vi "XYGraph.CreateErrorBars.vi"(0 "X":dbl[](array[numeric]) format="%.2f", 5 "Y":dbl[](array[numeric]) format="%.2f", 7 "error low":dbl[](array[numeric]) format="%.2f", 9 "error high":dbl[](array[numeric]) format="%.2f") -> (4 "xy graph bin 2":cluster{"X":dbl[], "Y":dbl[]}[](graph))   [LabVIEW 2013]
doc: "Creates a error bar plot\n\nwww.sciware.com.au"
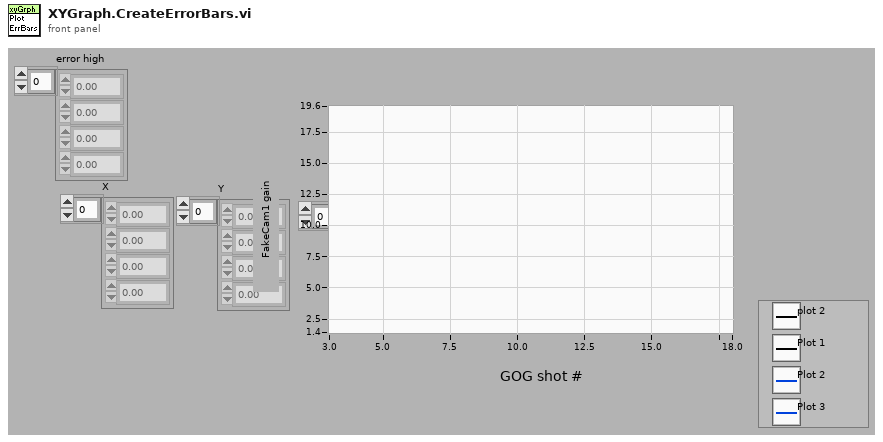
[diagram p1: front panel]
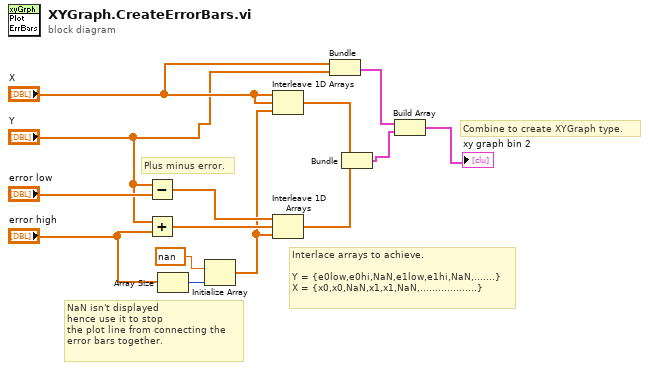
[diagram p0: block diagram]
diagram:
  # "Combine to create XYGraph type."
  # "Interlace arrays to achieve.\n\nY = {e0low,e0hi,NaN,e1low,e1hi,NaN,.......}\nX = {x0,x0,NaN,x1,x1,NaN,...................}"
  # "NaN isn't displayed\nhence use it to stop\nthe plot line from connecting the\nerror bars together."
  # "Plus minus error."
  n1 = Subtract(x="Y", y="error low") -> (x-y=w14:dbl[])
  n2 = Add(x="Y", y="error high") -> (x+y=w13:dbl[])
  n3 = Array Size(array="error high") -> (size(s)=w12:i32)
  n4 = Initialize Array(nan ("element"), w12) -> (w9:dbl[])
  n5 = Interleave 1D Arrays("X", "X", w9) -> (w8:dbl[])
  n6 = Interleave 1D Arrays(w14, w13, w9) -> (w7:dbl[])
  n7 = Bundle("X"="X", "Y"="Y") -> (w3:cluster{"X":dbl[], "Y":dbl[]})  [unwired: 1 out]
  n8 = Bundle(w8, w7) -> (w2:cluster{dbl[], dbl[]})  [unwired: 1 out]
  n9 = Build Array(w3, w2) -> (→"xy graph bin 2":cluster{"X":dbl[], "Y":dbl[]}[])
